vi "Launcher.vi"   [LabVIEW 2019]
uses:
  5bb4e541-9723-48ea-bc60-b36629f13927.vi
  00ce4967-b500-41ec-81df-ecff8b3ffe82.vi
  <vilib>/ErrorRing/Error Ring.xnode
  user32.dll
  TestBench/LoadApp.vi
  TestBench/TestBench/TestBench.lvclass
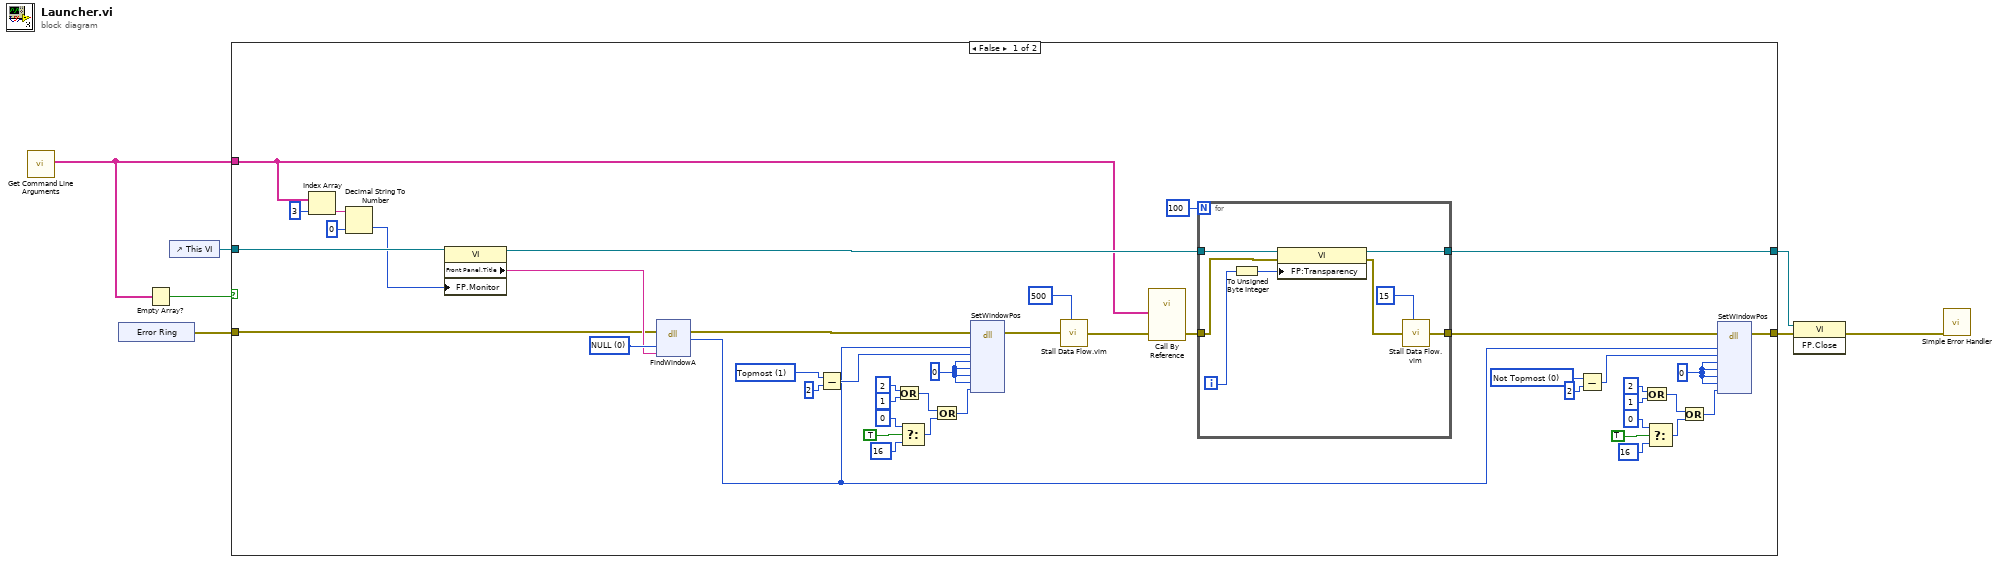
[diagram p0: block diagram]
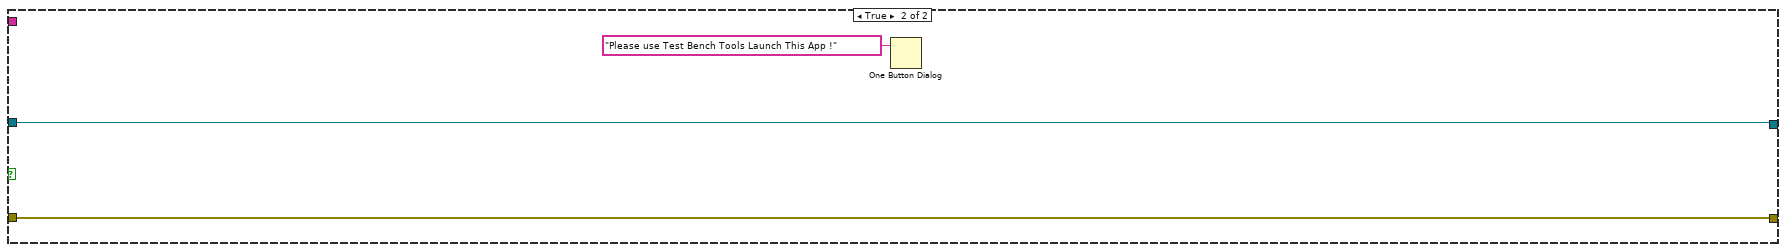
[diagram p2: hidden frame]
diagram:
  n1 = call <vilib>:"Get Command Line Arguments.vi"() -> ("arguments"=w4:string[])  [unwired: 9 in, 2 out]
  n2 = xnode "Error Ring"() -> ("error out"=w1:errorcluster)
  n3 = Empty Array?(array=w4) -> (empty?=w2:bool)
  n4 = control-ref of="This VI"() -> (w3:refnum<vi>)
  n5 = case shown="False" w2 {
    tunnel: [w49 w61] -> w7
    tunnel: [w17 w62] -> w6
    tunnel: w4 -> [w12 _]
    tunnel: w3 -> [w14 w61]
    tunnel: w1 -> [w13 w62]
    frame False {
      w19 = i16 0 items=["Not Topmost", "Topmost", "Top", "Bottom"] ("z-order position")
      w30 = 0
      w33 = i16 1 items=["Not Topmost", "Topmost", "Top", "Bottom"] ("z-order position")
      w44 = 0
      w45 = 0 items=["NULL"]
      n6 = Index Array(array=w12, index=3) -> (element=w10:string)
      n7 = Decimal String To Number(string=w10, default (0L)=u16 0 ("default (0 I32)")) -> (number=w8:u16)  [unwired: 1 in, 1 out]
      n8 = property class="VI"(reference=w14, "FP.Monitor"=w8) -> (reference out=w51:refnum<vi>, "Front Panel.Title"=w32:string)  [unwired: 1 in, 1 out]
      n9 = dll-call lib="user32.dll" fn="FindWindowA" label="FindWindow"(error in=w13, "lpszClassName"=w45, "lpszWindowName"=w32) -> (error out=w15:errorcluster, "hWnd"=w16:u32)  [unwired: 4 in, 1 out]
      n10 = Subtract(x=w33, y=i16 2) -> (x-y=w35:i16)
      n11 = Or(x=u32 2 ("SWP_NOMOVE"), y=u32 1 ("SWP_NOSIZE")) -> (x .or. y?=w42:u32)
      n12 = Select(t=u32 0, s=TRUE ("activate? (T)"), f=u32 16 ("SWP_NOACTIVATE")) -> (s? t:f=w41:u32)
      n13 = Or(x=w42, y=w41) -> (x .or. y?=w43:u32)
      n14 = dll-call lib="user32.dll" fn="SetWindowPos"(error in=w15, "hWnd"=w16, "hWndInsertAfter"=w35, "left"=w44, "top"=w44, "width"=w44, "height"=w44, "fuFlags"=w43) -> (error out=w31:errorcluster)  [unwired: 10 in, 1 out]
      n15 = call "Stall Data Flow.vim"("value in"=w31, "milliseconds to wait"=u32 500) -> ("value out"=w47:errorcluster)  [unwired: 1 out]
      n16 = call-by-ref "?"("error in (no error)"=w47, "arguments"=w12) -> ("error out"=w50:errorcluster)  [unwired: 11 in, 2 out]
      n17 = for {
        N: 100 -> [_]
        tunnel: w51 -> [w59]
        tunnel: w50 -> [w58]
        tunnel: [w57] -> w49
        tunnel: [w55] -> w18
        i -> [w53]
        n18 = To Unsigned Byte Integer(number=w53) -> (unsigned 8bit integer=w52:u8)
        n19 = property class="VI"(reference=w59, error in=w58, "FP:Transparency"=w52) -> (reference out=w57:refnum<vi>, error out=w56:errorcluster)
        n20 = call "Stall Data Flow.vim"("value in"=w56, "milliseconds to wait"=u32 15) -> ("value out"=w55:errorcluster)  [unwired: 1 out]
      }
      n21 = Subtract(x=w19, y=i16 2) -> (x-y=w21:i16)
      n22 = Or(x=u32 2 ("SWP_NOMOVE"), y=u32 1 ("SWP_NOSIZE")) -> (x .or. y?=w28:u32)
      n23 = Select(t=u32 0, s=TRUE ("activate? (T)"), f=u32 16 ("SWP_NOACTIVATE")) -> (s? t:f=w27:u32)
      n24 = Or(x=w28, y=w27) -> (x .or. y?=w29:u32)
      n25 = dll-call lib="USER32.DLL" fn="SetWindowPos"(error in=w18, "hWnd"=w16, "hWndInsertAfter"=w21, "left"=w30, "top"=w30, "width"=w30, "height"=w30, "fuFlags"=w29) -> (error out=w17:errorcluster)  [unwired: 10 in, 1 out]
    }
    frame True {
      n26 = One Button Dialog(message="Please use Test Bench Tools Launch This App !") -> ()  [unwired: 1 in, 1 out]
    }
  }
  n27 = invoke class="VI" method="FP.Close"(reference=w7, error in=w6) -> (error out=w5:errorcluster)  [unwired: 1 in, 2 out]
  n28 = call <vilib>:"Simple Error Handler.vi"("error in (no error)"=w5) -> ()  [unwired: 4 in, 5 out]
